vi "DriveStateController2.vi"(1 "Selected State (In)":string) -> (0 "Selected State (Out)":string)   [LabVIEW 2019]
doc: "This VI performs all of the calculations and decisions related to the swerve drive."
uses:
  dsinstructions.vi
  constants.vi
  dsdata.vi
  sensors.vi
  outputs.vi
panel:
  in  "Driver Profiles":T1(array[cluster])=[{"Strafe Deadband"=0.08, "Rotation Deadband"=0.15, "Strafe Scaling"=3.0, "Rotation Scaling"=2.5}, {"Strafe Deadband"=0.08, "Rotation Deadband"=0.15, "Strafe Scaling"=2.0, "Rotation Scaling"=2.5}, {"Strafe Deadband"=0.08, "Rotation Deadband"=0.15, "Strafe Scaling"=2.0, "Rotation Scaling"=2.5}, {"Strafe Deadband"=0.08, "Rotation Deadband"=0.15, "Strafe Scaling"=2.0, "Rotation Scaling"=2.5}] {"Rotation Scaling" min=1.0 max=4.0 scale=1.0..4.0; "Strafe Scaling" min=1.0 max=4.0 scale=1.0..4.0; "Rotation Deadband" min=0.0 max=0.4 scale=0.0..0.4; "Strafe Deadband" min=0.0 max=0.4 scale=0.0..0.4}
  out "Heading Control":bool
  in  "Heading Lock Strafe Deadband (ft/s)":dbl=2.0
  in  "PID Tuning Heading Lock":T2={"Kp"=0.007, "Ki"=0.03, "Kd"=0.0015, "N-Diff"=5, "N-Int"=10, "Int Error Window"=30.0, "Max Ouput"=1.0, "Min Output"=-1.0} {"Int Error Window" min=0.0; "N-Int" min=2; "N-Diff" min=2; "Kd" min=0.0; "Ki" min=0.0; "Kp" min=0.0}
  in  "Manually Disable Heading Lock":bool
  in  "PID Tuning Feeder Station":T2={"Kp"=0.01, "Ki"=0.01, "Kd"=9e-05, "N-Diff"=10, "N-Int"=10, "Int Error Window"=30.0, "Max Ouput"=1.0, "Min Output"=-1.0} {"Int Error Window" min=0.0; "N-Int" min=2; "N-Diff" min=2; "Kd" min=0.0; "Ki" min=0.0; "Kp" min=0.0}
  out "Heading Controller Summary":T3(graph)
  in  "PID Tuning Auto Targeting":T2={"Kp"=0.01, "Ki"=0.01, "Kd"=9e-05, "N-Diff"=10, "N-Int"=10, "Int Error Window"=30.0, "Max Ouput"=1.0, "Min Output"=-1.0} {"Int Error Window" min=0.0; "N-Int" min=2; "N-Diff" min=2; "Kd" min=0.0; "Ki" min=0.0; "Kp" min=0.0}
  in  "Manual Fudge Factor (deg)":dbl=5.0
  in  "Plot Heading PID":bool
  in  "Sync Driver Profile":bool
  out "Selected Driver":string
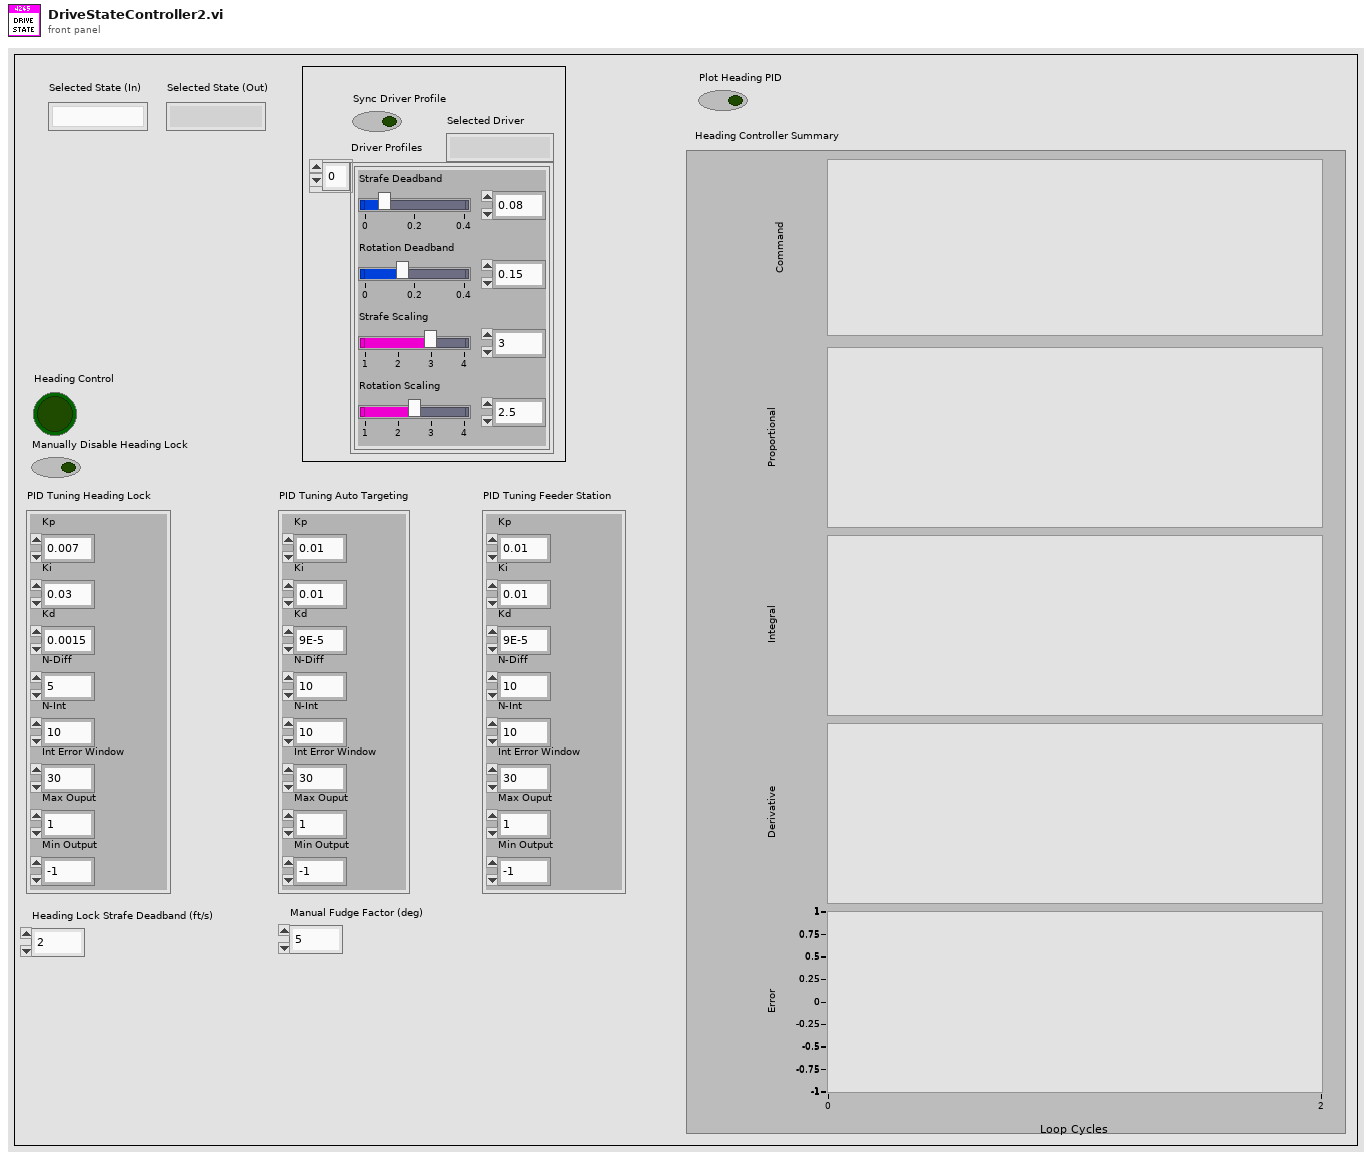
[diagram p1: front panel]
types:
  T1 = cluster{"Strafe Deadband":dbl, "Rotation Deadband":dbl, "Strafe Scaling":dbl, "Rotation Scaling":dbl}[]
  T2 = cluster{"Kp":dbl, "Ki":dbl, "Kd":dbl, "N-Diff":i32, "N-Int":i32, "Int Error Window":dbl, "Max Ouput":dbl, "Min Output":dbl}
  T3 = cluster{"Command":dbl, "Proportional":dbl, "Integral":dbl, "Derivative":dbl, "Goal":dbl}
  T4 = enum16{"Driver Control", "Auto Targeting", "Feeder Station"}
  T5 = cluster{"Strafe Deadband":dbl, "Rotation Deadband":dbl, "Strafe Scaling":dbl, "Rotation Scaling":dbl}
  T6 = enum16{"Center", "Module 0", "Module 1", "Module 2", "Module 3"}
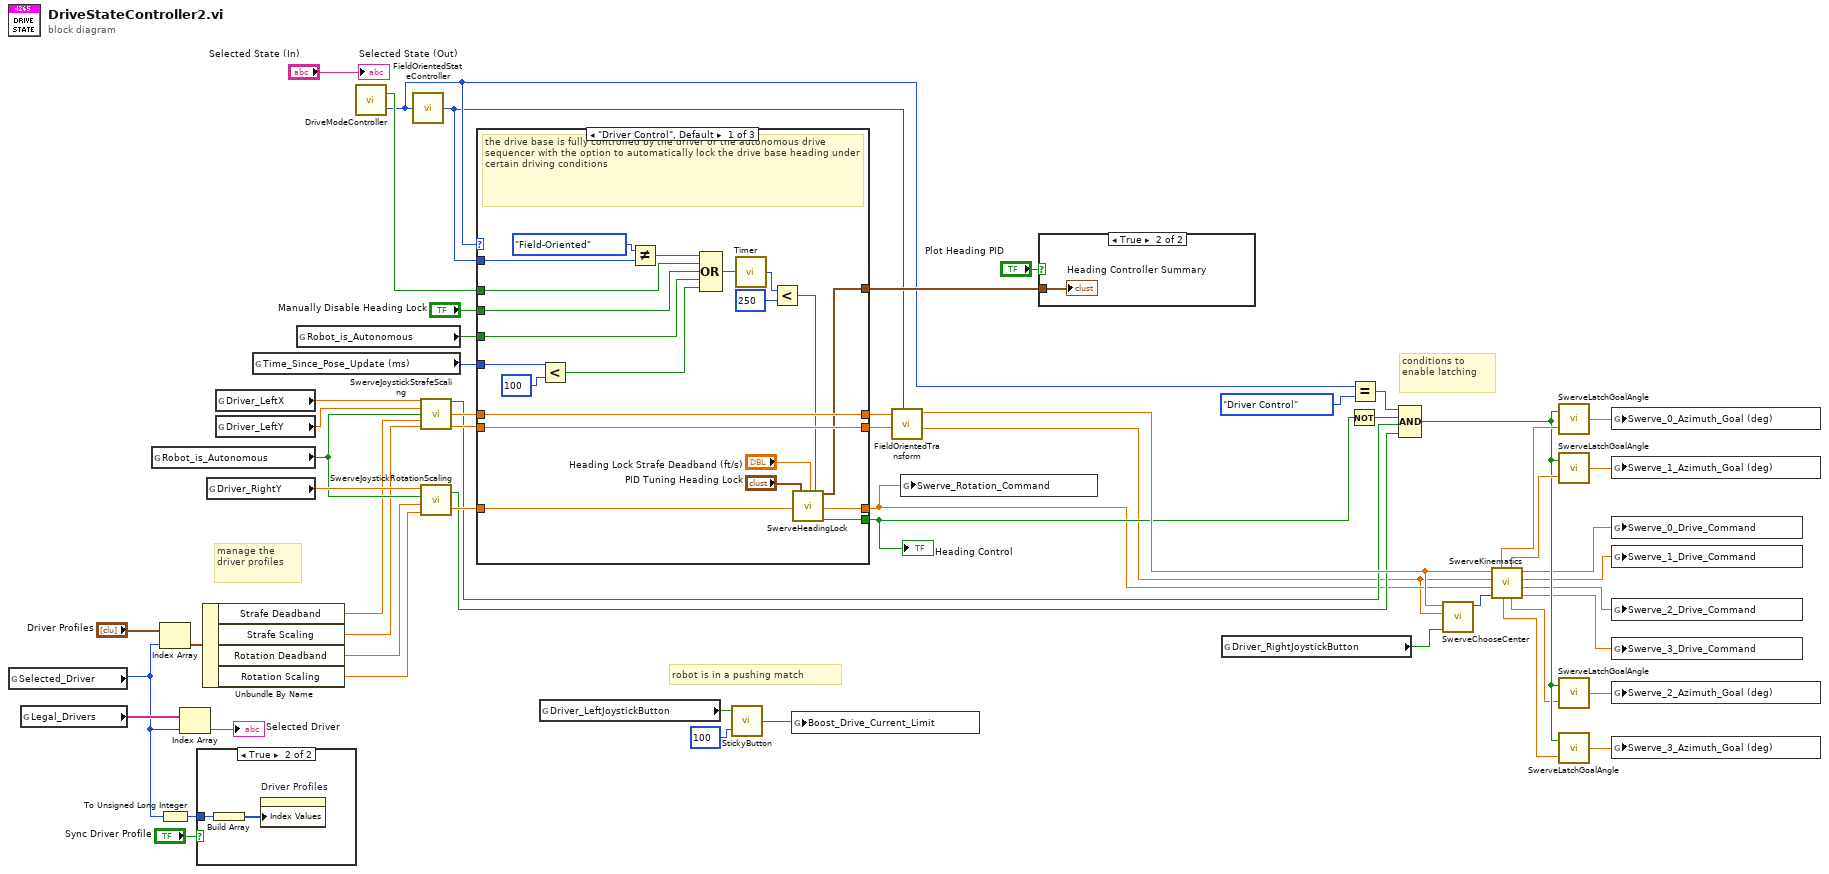
[diagram p0: block diagram]
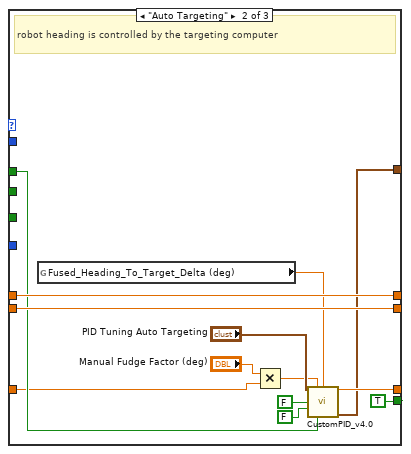
[diagram p3: hidden frame]
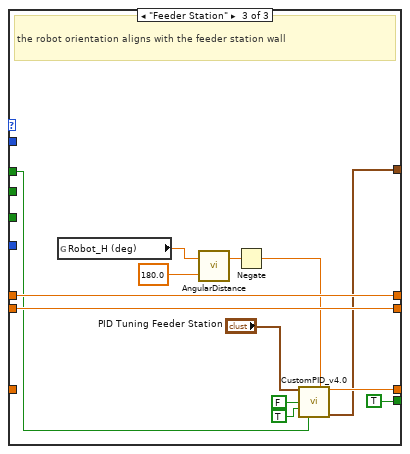
[diagram p4: hidden frame]
diagram:
  # "robot is in a pushing match"
  # "conditions to\nenable latching"
  # "manage the\ndriver profiles"
  n1 = global read "dsdata.vi" "Selected_Driver"() -> (w15:i32)
  n2 = global read "constants.vi" "Legal_Drivers"() -> (w50:string[])
  n3 = global read "dsdata.vi" "Robot_is_Autonomous"() -> (w29:bool)
  n4 = Index Array(array="Driver Profiles", index=w15) -> (element=w14:T5)
  n5 = To Unsigned Long Integer(number=w15) -> (unsigned 32bit integer=w52:u32)
  n6 = Index Array(array=w50, index=w15) -> (element=→"Selected Driver":string)
  n7 = case shown="True" "Sync Driver Profile" {
    tunnel: w52 -> [_ w58]
    frame False {
    }
    frame True {
      n8 = Build Array(w58) -> (w57:u32[])
      n9 = property on="Driver Profiles" class="Arr (strict)"("Index Values"=w57) -> ()  [unwired: 2 in, 2 out]
    }
  }
  n10 = Unbundle By Name(w14) -> ("Strafe Deadband"=w13:dbl, "Strafe Scaling"=w12:dbl, "Rotation Deadband"=w11:dbl, "Rotation Scaling"=w10:dbl)
  n11 = global read "dsinstructions.vi" "Driver_RightY"() -> (w30:dbl)
  n12 = global read "dsinstructions.vi" "Driver_LeftX"() -> (w35:dbl)
  n13 = global read "dsinstructions.vi" "Driver_LeftY"() -> (w34:dbl)
  n14 = global read "sensors.vi" "Time_Since_Pose_Update (ms)"() -> (w45:u32)
  n15 = global read "dsdata.vi" "Robot_is_Autonomous"() -> (w44:bool)
  n16 = call "DriveModeController.vi"() -> ("Drive Mode Change"=w42:bool, "Drive Mode"=w21:T4)  [unwired: 1 in]
  n17 = call "FieldOrientedStateController.vi"("Drive Mode"=w21) -> ("Orientation Mode"=w18:enum16{"Robot-Oriented", "Field-Oriented"})
  n18 = call "SwerveJoystickStrafeScaling.vi"("Raw Joystick X"=w35, "Raw Joystick Y"=w34, "Auto Control"=w29, "Strafe Deadband"=w13, "Strafe Scaling"=w12) -> ("In Deadband"=w25:bool, "Scaled Joystick X"=w33:dbl, "Scaled Joystick Y"=w32:dbl)  [unwired: 8 in]
  n19 = call "SwerveJoystickRotationScaling.vi"("Rotation Scaling"=w10, "Rotation Deadband"=w11, "Auto Control"=w29, "Raw Joystick Rotation"=w30) -> ("Scaled Joystick Rotation"=w31:dbl, "In Deadband"=w26:bool)
  n20 = case shown="\"Driver Control\", Default" w21 {
    tunnel: [w75 w91 w103] -> w17
    tunnel: [w74 w92 w101] -> w56
    tunnel: w33 -> [w74 w92 w101]
    tunnel: w32 -> [w75 w91 w103]
    tunnel: w31 -> [w67 w81 _]
    tunnel: [w68 w83 w100] -> w24
    tunnel: [w73 TRUE ("auto rot control") TRUE ("auto rot control")] -> w27
    tunnel: w18 -> [w76 _ _]
    tunnel: w44 -> [w71 _ _]
    tunnel: w42 -> [w64 w86 w96]
    tunnel: w45 -> [w79 _ _]
    tunnel: [w70 w82 w95] -> w43
    tunnel: "Manually Disable Heading Lock" -> [w69 _ _]
    frame "Driver Control", Default {
      # "the drive base is fully controlled by the driver or the autonomous drive sequencer with the option to automatically lock the drive base heading under certain driving conditions"
      n21 = Less?(x=w79, y=u32 100) -> (x < y?=w72:bool)
      n22 = Not Equal?(x=enum16{"Robot-Oriented", "Field-Oriented"}."Field-Oriented" ("Orientation Mode"), y=w76) -> (x != y?=w63:bool)
      n23 = Compound Arithmetic op=OR(w63, w64, w69, w71, w72) -> (w61:bool)
      n24 = call "Timer.vi"("Reset Timer"=w61) -> ("Time (ms)"=w62:u32)
      n25 = Less?(x=w62, y=u32 250) -> (x < y?=w59:bool)
      n26 = call "SwerveHeadingLock.vi"("Driver Rotation Joystick"=w67, "PID Tuning Parameters"="PID Tuning Heading Lock", "Heading Lock Strafe Deadband (ft/s)"="Heading Lock Strafe Deadband (ft/s)", "External Disables"=w59) -> ("Controller Summary"=w70:T3, "Joystick Rotation"=w68:dbl, "Heading Lock"=w73:bool)  [unwired: 13 in]
    }
    frame "Auto Targeting" {
      # "robot heading is controlled by the targeting computer"
      n27 = global read "sensors.vi" "Fused_Heading_To_Target_Delta (deg)"() -> (w87:dbl)
      n28 = Multiply(x="Manual Fudge Factor (deg)", y=w81) -> (x*y=w88:dbl)
      n29 = call "CustomPID_v4.0.vi"("PID Tuning Parameters"="PID Tuning Auto Targeting", "Goal"=w88, "Process Variable"=w87, "Reset on Goal Change ?"=FALSE, "Use Custom Error Calculation ?"=FALSE, "Reinit"=w86) -> ("Command"=w83:dbl, "Controller Summary"=w82:T3)  [unwired: 6 in, 2 out]
    }
    frame "Feeder Station" {
      # "the robot orientation aligns with the feeder station wall"
      n30 = global read "sensors.vi" "Robot_H (deg)"() -> (w105:dbl)
      n31 = call "AngularDistance.vi"("Goal Angle (deg) [0,360]"=180.0, "Current Angle (deg) [-Inf,+Inf]"=w105) -> ("Signed Angular Distance (deg) [-180,+180]"=w94:dbl)  [unwired: 1 out]
      n32 = Negate(x=w94) -> (-x=w93:dbl)
      n33 = call "CustomPID_v4.0.vi"("PID Tuning Parameters"="PID Tuning Feeder Station", "Custom Error Calculation"=w93, "Reset on Goal Change ?"=FALSE, "Use Custom Error Calculation ?"=TRUE, "Reinit"=w96) -> ("Command"=w100:dbl, "Controller Summary"=w95:T3)  [unwired: 7 in, 2 out]
    }
  }
  "Heading Control" <- w27
  n34 = global read "dsinstructions.vi" "Driver_LeftJoystickButton"() -> (w38:bool)
  n35 = call "StickyButton.vi"("Time threshold (ms)"=u32 100 ("y"), "Button Input"=w38) -> ("Sticky Button"=w36:bool)
  n36 = global write "outputs.vi" "Boost_Drive_Current_Limit"(w36) -> ()
  n37 = call "FieldOrientedTransform.vi"("Orientation Mode"=w18, "Joystick Y"=w17, "Joystick X"=w56) -> ("Joystick Y'"=w19:dbl, "Joystick X'"=w28:dbl)  [unwired: 7 in]
  n38 = global write "outputs.vi" "Swerve_Rotation_Command"(w24) -> ()
  n39 = case shown="True" "Plot Heading PID" {
    tunnel: w43 -> [_ w106]
    frame False {
    }
    frame True {
      "Heading Controller Summary" <- w106
    }
  }
  n40 = global read "dsinstructions.vi" "Driver_RightJoystickButton"() -> (w41:bool)
  n41 = Not(x=w27) -> (.not. x?=w23:bool)
  n42 = Equal?(x=w21, y=T4."Driver Control" ("x")) -> (x = y?=w22:bool)
  n43 = Compound Arithmetic op=AND(w22, w23, w25, w26) -> (w48:bool)
  n44 = call "SwerveChooseCenter.vi"("Defensive Driving Trigger"=w41, "Joystick Y"=w19, "Joystick X"=w28) -> ("Center Choice"=w40:T6)  [unwired: 6 in]
  n45 = call "SwerveKinematics.vi"("Rotation Center Choice"=w40, "Joystick Rotation"=w24, "Joystick Y"=w19, "Joystick X"=w28) -> ("Module 3 Velocity Command (ul)"=w5:dbl, "Module 2 Velocity Command (ul)"=w6:dbl, "Module 1 Velocity Command (ul)"=w7:dbl, "Module 0 Velocity Command (ul)"=w8:dbl, "Module 2 Angle (deg)"=w47:dbl, "Module 1 Angle (deg)"=w54:dbl, "Module 3 Angle (deg)"=w46:dbl, "Module 0 Angle (deg)"=w55:dbl)
  n46 = call "SwerveLatchGoalAngle.vi"("Raw Goal Angle"=w55, "In Deadband"=w48) -> ("Latched Goal Angle"=w4:dbl)
  n47 = call "SwerveLatchGoalAngle.vi"("Raw Goal Angle"=w54, "In Deadband"=w48) -> ("Latched Goal Angle"=w3:dbl)
  n48 = call "SwerveLatchGoalAngle.vi"("Raw Goal Angle"=w47, "In Deadband"=w48) -> ("Latched Goal Angle"=w2:dbl)
  n49 = call "SwerveLatchGoalAngle.vi"("Raw Goal Angle"=w46, "In Deadband"=w48) -> ("Latched Goal Angle"=w1:dbl)
  n50 = global write "outputs.vi" "Swerve_0_Azimuth_Goal (deg)"(w4) -> ()
  n51 = global write "outputs.vi" "Swerve_1_Azimuth_Goal (deg)"(w3) -> ()
  n52 = global write "outputs.vi" "Swerve_0_Drive_Command"(w8) -> ()
  n53 = global write "outputs.vi" "Swerve_1_Drive_Command"(w7) -> ()
  n54 = global write "outputs.vi" "Swerve_2_Drive_Command"(w6) -> ()
  n55 = global write "outputs.vi" "Swerve_3_Drive_Command"(w5) -> ()
  n56 = global write "outputs.vi" "Swerve_2_Azimuth_Goal (deg)"(w2) -> ()
  n57 = global write "outputs.vi" "Swerve_3_Azimuth_Goal (deg)"(w1) -> ()
  "Selected State (Out)" <- "Selected State (In)"
